vi "Configure Math Function.vi"(6 "Operation (0: Add)":T1(ring), 7 "Channel (T: Enable)":bool=TRUE, 8 "error in (no error)":errorcluster, 9 "Source2 (1: Channel 2)":u16(ring)=1 items=["Channel 1", "Channel 2", "Channel 3", "Channel 4"], 10 "Source1 (0: Channel 1)":u16(ring) items=["Channel 1", "Channel 2", "Channel 3", "Channel 4", "g( t )"], 11 "VISA resource name":refnum<visa-resource-name>) -> (0 "error out":errorcluster, 3 "VISA resource name out":refnum<visa-resource-name>)   [LabVIEW 2017, in "Agilent 6000 Series.lvlib"]
doc: "This VI configures the properties that control the math channel. These properties are the sources and operation."
uses:
  <instrlib>/Agilent 6000 Series/Agilent 6000 Series.lvlib
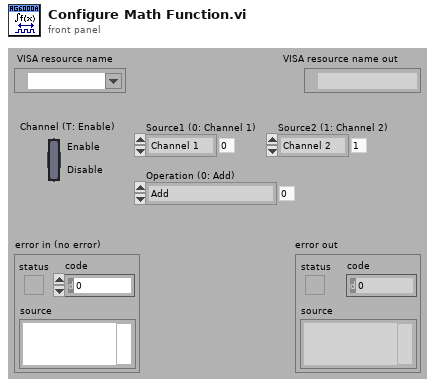
[diagram p1: front panel]
types:
  T1 = enum16{"Add", "Subtract", "Multiply", "Integrate", "Differentiate", "FFT", "Square Root", "g( t ): Source1 + Source2", "g( t ): Source1 - Source2", "g( t ): Source1 * Source2"}
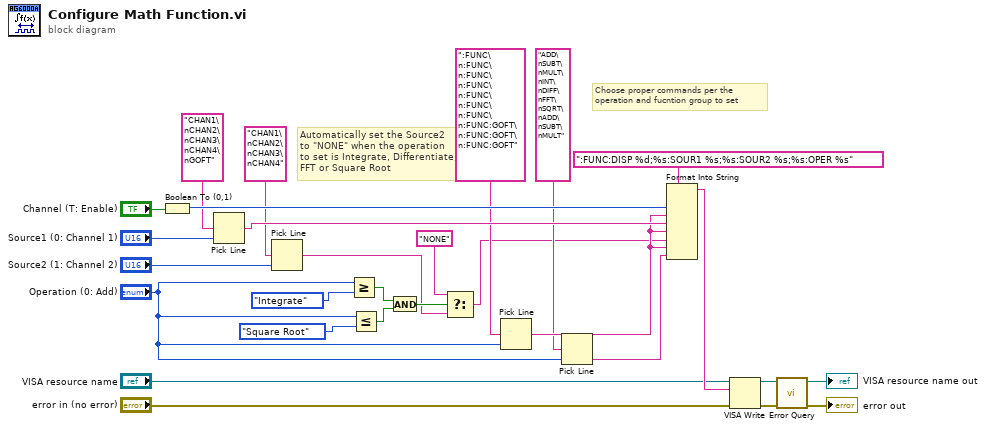
[diagram p0: block diagram]
diagram:
  # "Choose proper commands per the\noperation and fucntion group to set"
  # "Automatically set the Source2\nto \"NONE\" when the operation\nto set is Integrate, Differentiate,\nFFT or Square Root"
  n1 = Boolean To (0,1)(Boolean="Channel (T: Enable)") -> (0, 1=w26:i16)
  n2 = Pick Line(multi-line string="CHAN1\nCHAN2\nCHAN3\nCHAN4\nGOFT", line index="Source1 (0: Channel 1)") -> (output string=w24:string)  [unwired: 1 in]
  n3 = Pick Line(multi-line string="CHAN1\nCHAN2\nCHAN3\nCHAN4", line index="Source2 (1: Channel 2)") -> (output string=w4:string)  [unwired: 1 in]
  n4 = Greater Or Equal?(x="Operation (0: Add)", y=T1."Integrate") -> (x >= y?=w7:bool)
  n5 = Less Or Equal?(x="Operation (0: Add)", y=T1."Square Root") -> (x <= y?=w8:bool)
  n6 = And(x=w7, y=w8) -> (x .and. y?=w6:bool)
  n7 = Select(t="NONE", s=w6, f=w4) -> (s? t:f=w3:string)
  n8 = Pick Line(multi-line string=":FUNC\n:FUNC\n:FUNC\n:FUNC\n:FUNC\n:FUNC\n:FUNC\n:FUNC:GOFT\n:FUNC:GOFT\n:FUNC:GOFT", line index="Operation (0: Add)") -> (output string=w21:string)  [unwired: 1 in]
  n9 = Pick Line(multi-line string="ADD\nSUBT\nMULT\nINT\nDIFF\nFFT\nSQRT\nADD\nSUBT\nMULT", line index="Operation (0: Add)") -> (output string=w17:string)  [unwired: 1 in]
  n10 = Format Into String(format string=":FUNC:DISP %d;%s:SOUR1 %s;%s:SOUR2 %s;%s:OPER %s", w26, w21, w24, w21, w3, w21, w17) -> (resulting string=w16:string)  [unwired: 2 in, 1 out]
  n11 = VISA Write(VISA resource name="VISA resource name", write buffer=w16, error in (no error)="error in (no error)") -> (VISA resource name out=w11:refnum<visa-resource-name>, error out=w10:errorcluster)  [unwired: 1 out]
  n12 = call <instrlib>:"Error Query.vi"("error in (no error)"=w10, "VISA resource name"=w11) -> ("error out"=→"error out":errorcluster, "VISA resource name out"=→"VISA resource name out":refnum<visa-resource-name>)  [unwired: 6 in, 2 out]
